vi "XML toTestSetDef.vi"(11 "TSD XML":string) -> (3 "Test Set Definition":T1={"General"={"ID"=0, "Model"="", "Dual Port?"=FALSE, "Options"="", "Options"={"E"=FALSE, "K"=FALSE, "H"=FALSE, "W"=FALSE, "F"=FALSE}, "Cal File"=path ""}, "Receiver"={"Fstart, MHz"=0.0, "Fstop MHz"=0.0, "Fstep MHz"=0.0, "IF, MHz"=0.0}, "RX Band"={"Fstart, MHz"=0.0, "Fstop MHz"=0.0}, "TX 1"={"Fstart, MHz"=0.0, "Fstop MHz"=0.0, "Pmax, dBm"=0.0, "Pstep, dB"=0.0}, "TX 2"={"Fstart, MHz"=0.0, "Fstop MHz"=0.0, "Pmax, dBm"=0.0, "Pstep, dB"=0.0}, "Low-side?"=TRUE})   [LabVIEW 2011]
uses:
  Test Set Definition.ctl
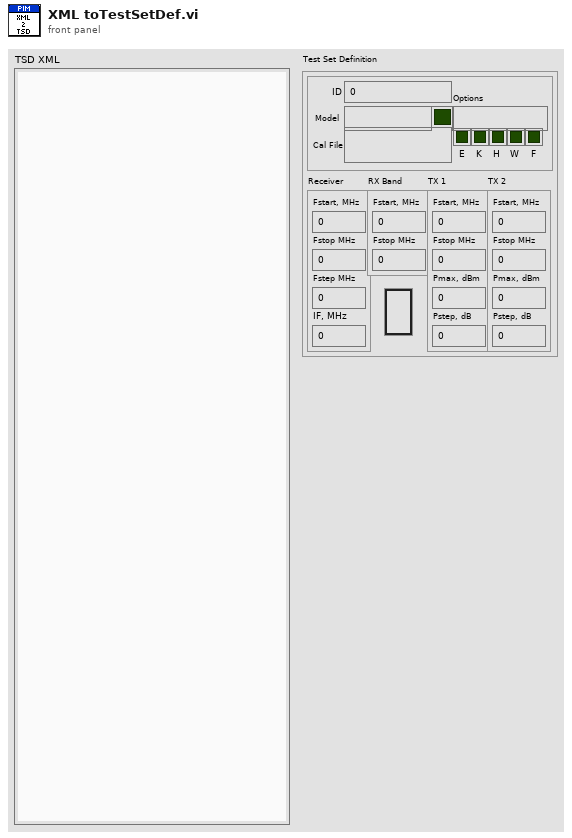
[diagram p1: front panel]
types:
  T1 = typedef "Test Set Definition.ctl" = cluster{"General":cluster{"ID":u32, "Model":string, "Dual Port?":bool, "Options":string, "Options":cluster{"E":bool, "K":bool, "H":bool, "W":bool, "F":bool}, "Cal File":path}, "Receiver":cluster{"Fstart, MHz":dbl, "Fstop MHz":dbl, "Fstep MHz":dbl, "IF, MHz":dbl}, "RX Band":cluster{"Fstart, MHz":dbl, "Fstop MHz":dbl}, "TX 1":cluster{"Fstart, MHz":dbl, "Fstop MHz":dbl, "Pmax, dBm":dbl, "Pstep, dB":dbl}, "TX 2":cluster{"Fstart, MHz":dbl, "Fstop MHz":dbl, "Pmax, dBm":dbl, "Pstep, dB":dbl}, "Low-side?":bool}
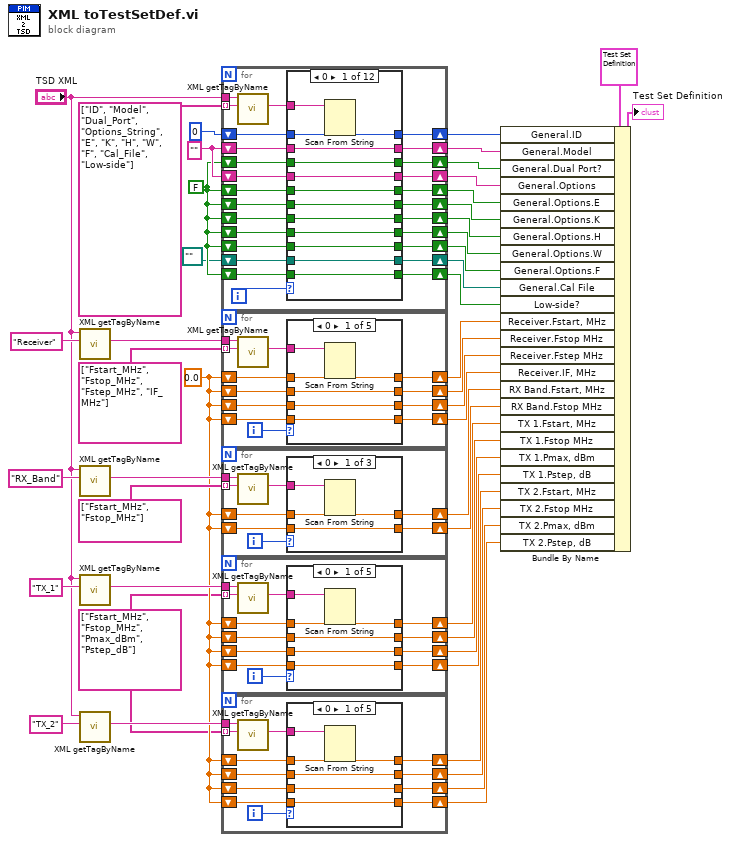
[diagram p0: block diagram]
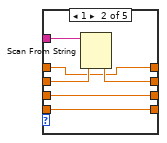
[diagram p2: hidden frame]
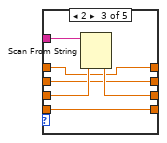
[diagram p3: hidden frame]
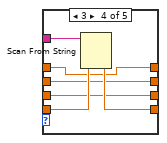
[diagram p4: hidden frame]
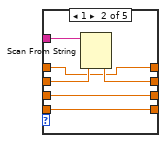
[diagram p6: hidden frame]
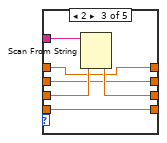
[diagram p7: hidden frame]
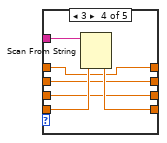
[diagram p8: hidden frame]
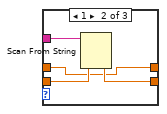
[diagram p10: hidden frame]
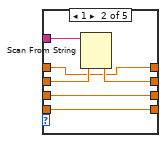
[diagram p12: hidden frame]
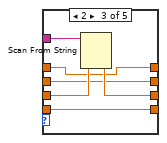
[diagram p13: hidden frame]
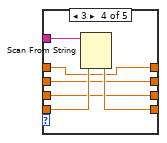
[diagram p14: hidden frame]
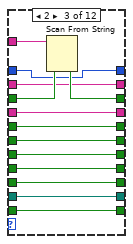
[diagram p17: hidden frame]
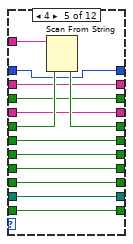
[diagram p19: hidden frame]
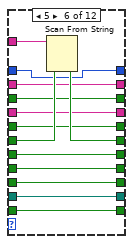
[diagram p20: hidden frame]
diagram:
  w10 = string[] ["Fstart_MHz", "Fstop_MHz", "Pmax_dBm", "Pstep_dB"]
  w11 = 0.0 ("General.ID")
  w40 = FALSE
  w41 = "" ("General.Model")
  n1 = call "XML getTagByName.vi"("Tag Name"="Receiver", "XML String"="TSD XML") -> ("Tag Contents"=w25:string)  [unwired: 5 in, 4 out]
  n2 = call "XML getTagByName.vi"("Tag Name"="RX_Band", "XML String"="TSD XML") -> ("Tag Contents"=w24:string)  [unwired: 5 in, 4 out]
  n3 = call "XML getTagByName.vi"("Tag Name"="TX_1", "XML String"="TSD XML") -> ("Tag Contents"=w20:string)  [unwired: 5 in, 4 out]
  n4 = call "XML getTagByName.vi"("Tag Name"="TX_2", "XML String"="TSD XML") -> ("Tag Contents"=w19:string)  [unwired: 5 in, 4 out]
  n5 = for {
    tunnel: string[] ["ID", "Model", "Dual_Port", "Options_String", "E", "K", "H", "W", "F", "Cal_File", "Low-side"] -> [w71] mode=indexing
    shift-right: [w56] -> w38
    shift-left: u32 0 ("General.ID") -> [w59]
    shift-right: [w55] -> w37
    shift-left: w41 -> [w60]
    shift-right: [w54] -> w36
    shift-left: w40 -> [w61]
    shift-right: [w53] -> w35
    shift-left: w41 -> [w62]
    shift-right: [w52] -> w34
    shift-left: w40 -> [w63]
    shift-right: [w51] -> w33
    shift-left: w40 -> [w64]
    shift-right: [w50] -> w32
    shift-left: w40 -> [w65]
    shift-right: [w49] -> w31
    shift-left: w40 -> [w66]
    shift-right: [w48] -> w30
    shift-left: w40 -> [w67]
    shift-right: [w47] -> w29
    shift-left: path "" ("General.Cal File") -> [w68]
    shift-right: [w46] -> w28
    shift-left: w40 -> [w69]
    tunnel: "TSD XML" -> [w70]
    i -> [w58]
    n6 = call "XML getTagByName.vi"("Tag Name"=w71, "XML String"=w70) -> ("Tag Contents"=w57:string)  [unwired: 5 in, 4 out]
    n7 = case shown="0" w58 {
      tunnel: w69 -> [w72 w86 w96 w110 w120 w133 w146 w159 w172 w185 w209 w212]
      tunnel: w68 -> [w73 w87 w97 w111 w121 w134 w147 w160 w173 w196 w198 w213]
      tunnel: w67 -> [w74 w88 w98 w112 w122 w135 w148 w161 w183 w186 w199 w214]
      tunnel: w66 -> [w75 w89 w99 w113 w123 w136 w149 w170 w174 w187 w200 w215]
      tunnel: w65 -> [w76 w90 w100 w114 w124 w137 w157 w162 w175 w188 w201 w216]
      tunnel: w64 -> [w77 w91 w101 w115 w125 w144 w150 w163 w176 w189 w202 w217]
      tunnel: w63 -> [w78 w92 w102 w116 w131 w138 w151 w164 w177 w190 w203 w218]
      tunnel: w62 -> [w79 w93 w103 _ w126 w139 w152 w165 w178 w191 w204 w219]
      tunnel: w61 -> [w80 w94 w107 w117 w127 w140 w153 w166 w179 w192 w205 w220]
      tunnel: w60 -> [w81 _ w104 w118 w128 w141 w154 w167 w180 w193 w206 w221]
      tunnel: w59 -> [w83 w95 w105 w119 w129 w142 w155 w168 w181 w194 w207 w211]
      tunnel: w57 -> [w84 w85 w108 w109 w132 w145 w158 w171 w184 w197 w210 _]
      tunnel: [w82 w95 w105 w119 w129 w142 w155 w168 w181 w194 w207 w211] -> w56
      tunnel: [w81 w85 w104 w118 w128 w141 w154 w167 w180 w193 w206 w221] -> w55
      tunnel: [w80 w94 w106 w117 w127 w140 w153 w166 w179 w192 w205 w220] -> w54
      tunnel: [w79 w93 w103 w109 w126 w139 w152 w165 w178 w191 w204 w219] -> w53
      tunnel: [w78 w92 w102 w116 w130 w138 w151 w164 w177 w190 w203 w218] -> w52
      tunnel: [w77 w91 w101 w115 w125 w143 w150 w163 w176 w189 w202 w217] -> w51
      tunnel: [w76 w90 w100 w114 w124 w137 w156 w162 w175 w188 w201 w216] -> w50
      tunnel: [w75 w89 w99 w113 w123 w136 w149 w169 w174 w187 w200 w215] -> w49
      tunnel: [w74 w88 w98 w112 w122 w135 w148 w161 w182 w186 w199 w214] -> w48
      tunnel: [w73 w87 w97 w111 w121 w134 w147 w160 w173 w195 w198 w213] -> w47
      tunnel: [w72 w86 w96 w110 w120 w133 w146 w159 w172 w185 w208 w212] -> w46
      frame 0 {
        n8 = Scan From String(input string=w84, default 1=w83) -> (output 1=w82:u32)  [unwired: 3 in, 3 out]
      }
      frame 1 {
      }
      frame 2 {
        n9 = Scan From String(input string=w108, default 1=w107) -> (output 1=w106:bool)  [unwired: 3 in, 3 out]
      }
      frame 3 {
      }
      frame 4 {
        n10 = Scan From String(input string=w132, default 1=w131) -> (output 1=w130:bool)  [unwired: 3 in, 3 out]
      }
      frame 5 {
        n11 = Scan From String(input string=w145, default 1=w144) -> (output 1=w143:bool)  [unwired: 3 in, 3 out]
      }
      frame 6 {
        n12 = Scan From String(input string=w158, default 1=w157) -> (output 1=w156:bool)  [unwired: 3 in, 3 out]
      }
      frame 7 {
        n13 = Scan From String(input string=w171, default 1=w170) -> (output 1=w169:bool)  [unwired: 3 in, 3 out]
      }
      frame 8 {
        n14 = Scan From String(input string=w184, default 1=w183) -> (output 1=w182:bool)  [unwired: 3 in, 3 out]
      }
      frame 9 {
        n15 = Scan From String(input string=w197, default 1=w196) -> (output 1=w195:path)  [unwired: 3 in, 3 out]
      }
      frame 10 {
        n16 = Scan From String(input string=w210, default 1=w209) -> (output 1=w208:bool)  [unwired: 3 in, 3 out]
      }
      frame Default {
      }
    }
  }
  n17 = for {
    tunnel: string[] ["Fstart_MHz", "Fstop_MHz", "Fstep_MHz", "IF_MHz"] -> [w233] mode=indexing
    shift-right: [w226] -> w17
    shift-left: w11 -> [w229]
    shift-right: [w225] -> w16
    shift-left: w11 -> [w230]
    shift-right: [w224] -> w15
    shift-left: w11 -> [w231]
    shift-right: [w223] -> w14
    shift-left: w11 -> [w232]
    tunnel: w25 -> [w222]
    i -> [w228]
    n18 = call "XML getTagByName.vi"("Tag Name"=w233, "XML String"=w222) -> ("Tag Contents"=w227:string)  [unwired: 5 in, 4 out]
    n19 = case shown="0" w228 {
      tunnel: w232 -> [w234 w240 w246 w256 w259]
      tunnel: w231 -> [w235 w241 w250 w252 w260]
      tunnel: w230 -> [w236 w244 w247 w253 w261]
      tunnel: w229 -> [w238 w242 w248 w254 w258]
      tunnel: w227 -> [w239 w245 w251 w257 _]
      tunnel: [w237 w242 w248 w254 w258] -> w226
      tunnel: [w236 w243 w247 w253 w261] -> w225
      tunnel: [w235 w241 w249 w252 w260] -> w224
      tunnel: [w234 w240 w246 w255 w259] -> w223
      frame 0 {
        n20 = Scan From String(input string=w239, default 1=w238) -> (output 1=w237:dbl)  [unwired: 3 in, 3 out]
      }
      frame 1 {
        n21 = Scan From String(input string=w245, default 1=w244) -> (output 1=w243:dbl)  [unwired: 3 in, 3 out]
      }
      frame 2 {
        n22 = Scan From String(input string=w251, default 1=w250) -> (output 1=w249:dbl)  [unwired: 3 in, 3 out]
      }
      frame 3 {
        n23 = Scan From String(input string=w257, default 1=w256) -> (output 1=w255:dbl)  [unwired: 3 in, 3 out]
      }
      frame Default {
      }
    }
  }
  n24 = for {
    tunnel: string[] ["Fstart_MHz", "Fstop_MHz"] -> [w269] mode=indexing
    shift-right: [w264] -> w13
    shift-left: w11 -> [w267]
    shift-right: [w263] -> w12
    shift-left: w11 -> [w268]
    tunnel: w24 -> [w262]
    i -> [w266]
    n25 = call "XML getTagByName.vi"("Tag Name"=w269, "XML String"=w262) -> ("Tag Contents"=w265:string)  [unwired: 5 in, 4 out]
    n26 = case shown="0" w266 {
      tunnel: w268 -> [w270 w276 w279]
      tunnel: w267 -> [w272 w274 w278]
      tunnel: w265 -> [w273 w277 _]
      tunnel: [w271 w274 w278] -> w264
      tunnel: [w270 w275 w279] -> w263
      frame 0 {
        n27 = Scan From String(input string=w273, default 1=w272) -> (output 1=w271:dbl)  [unwired: 3 in, 3 out]
      }
      frame 1 {
        n28 = Scan From String(input string=w277, default 1=w276) -> (output 1=w275:dbl)  [unwired: 3 in, 3 out]
      }
      frame Default {
      }
    }
  }
  n29 = for {
    tunnel: w10 -> [w291] mode=indexing
    shift-right: [w284] -> w9
    shift-left: w11 -> [w287]
    shift-right: [w283] -> w8
    shift-left: w11 -> [w288]
    shift-right: [w282] -> w7
    shift-left: w11 -> [w289]
    shift-right: [w281] -> w6
    shift-left: w11 -> [w290]
    tunnel: w20 -> [w280]
    i -> [w286]
    n30 = call "XML getTagByName.vi"("Tag Name"=w291, "XML String"=w280) -> ("Tag Contents"=w285:string)  [unwired: 5 in, 4 out]
    n31 = case shown="0" w286 {
      tunnel: w290 -> [w292 w298 w304 w314 w317]
      tunnel: w289 -> [w293 w299 w308 w310 w318]
      tunnel: w288 -> [w294 w302 w305 w311 w319]
      tunnel: w287 -> [w296 w300 w306 w312 w316]
      tunnel: w285 -> [w297 w303 w309 w315 _]
      tunnel: [w295 w300 w306 w312 w316] -> w284
      tunnel: [w294 w301 w305 w311 w319] -> w283
      tunnel: [w293 w299 w307 w310 w318] -> w282
      tunnel: [w292 w298 w304 w313 w317] -> w281
      frame 0 {
        n32 = Scan From String(input string=w297, default 1=w296) -> (output 1=w295:dbl)  [unwired: 3 in, 3 out]
      }
      frame 1 {
        n33 = Scan From String(input string=w303, default 1=w302) -> (output 1=w301:dbl)  [unwired: 3 in, 3 out]
      }
      frame 2 {
        n34 = Scan From String(input string=w309, default 1=w308) -> (output 1=w307:dbl)  [unwired: 3 in, 3 out]
      }
      frame 3 {
        n35 = Scan From String(input string=w315, default 1=w314) -> (output 1=w313:dbl)  [unwired: 3 in, 3 out]
      }
      frame Default {
      }
    }
  }
  n36 = for {
    tunnel: w10 -> [w331] mode=indexing
    shift-right: [w324] -> w5
    shift-left: w11 -> [w327]
    shift-right: [w323] -> w4
    shift-left: w11 -> [w328]
    shift-right: [w322] -> w3
    shift-left: w11 -> [w329]
    shift-right: [w321] -> w2
    shift-left: w11 -> [w330]
    tunnel: w19 -> [w320]
    i -> [w326]
    n37 = call "XML getTagByName.vi"("Tag Name"=w331, "XML String"=w320) -> ("Tag Contents"=w325:string)  [unwired: 5 in, 4 out]
    n38 = case shown="0" w326 {
      tunnel: w330 -> [w332 w338 w344 w354 w357]
      tunnel: w329 -> [w333 w339 w348 w350 w358]
      tunnel: w328 -> [w334 w342 w345 w351 w359]
      tunnel: w327 -> [w336 w340 w346 w352 w356]
      tunnel: w325 -> [w337 w343 w349 w355 _]
      tunnel: [w335 w340 w346 w352 w356] -> w324
      tunnel: [w334 w341 w345 w351 w359] -> w323
      tunnel: [w333 w339 w347 w350 w358] -> w322
      tunnel: [w332 w338 w344 w353 w357] -> w321
      frame 0 {
        n39 = Scan From String(input string=w337, default 1=w336) -> (output 1=w335:dbl)  [unwired: 3 in, 3 out]
      }
      frame 1 {
        n40 = Scan From String(input string=w343, default 1=w342) -> (output 1=w341:dbl)  [unwired: 3 in, 3 out]
      }
      frame 2 {
        n41 = Scan From String(input string=w349, default 1=w348) -> (output 1=w347:dbl)  [unwired: 3 in, 3 out]
      }
      frame 3 {
        n42 = Scan From String(input string=w355, default 1=w354) -> (output 1=w353:dbl)  [unwired: 3 in, 3 out]
      }
      frame Default {
      }
    }
  }
  n43 = Bundle By Name(cluster=T1 {"General"={"ID"=0, "Model"="", "Dual Port?"=FALSE, "Options"="", "Options"={"E"=FALSE, "K"=FALSE, "H"=FALSE, "W"=FALSE, "F"=FALSE}, "Cal File"=path ""}, "Receiver"={"Fstart, MHz"=0.0, "Fstop MHz"=0.0, "Fstep MHz"=0.0, "IF, MHz"=0.0}, "RX Band"={"Fstart, MHz"=0.0, "Fstop MHz"=0.0}, "TX 1"={"Fstart, MHz"=0.0, "Fstop MHz"=0.0, "Pmax, dBm"=0.0, "Pstep, dB"=0.0}, "TX 2"={"Fstart, MHz"=0.0, "Fstop MHz"=0.0, "Pmax, dBm"=0.0, "Pstep, dB"=0.0}, "Low-side?"=TRUE} ("Test Set Definition"), "General.ID"=w38, "General.Model"=w37, "General.Dual Port?"=w36, "General.Options"=w35, "General.Options.E"=w34, "General.Options.K"=w33, "General.Options.H"=w32, "General.Options.W"=w31, "General.Options.F"=w30, "General.Cal File"=w29, "Low-side?"=w28, "Receiver.Fstart, MHz"=w17, "Receiver.Fstop MHz"=w16, "Receiver.Fstep MHz"=w15, "Receiver.IF, MHz"=w14, "RX Band.Fstart, MHz"=w13, "RX Band.Fstop MHz"=w12, "TX 1.Fstart, MHz"=w9, "TX 1.Fstop MHz"=w8, "TX 1.Pmax, dBm"=w7, "TX 1.Pstep, dB"=w6, "TX 2.Fstart, MHz"=w5, "TX 2.Fstop MHz"=w4, "TX 2.Pmax, dBm"=w3, "TX 2.Pstep, dB"=w2) -> (→"Test Set Definition":T1)
